vi "Test_Sumadores_Javi.vi"(8 "error in (no error)":errorcluster, 9 "QR":string, 10 "Path":path, 11 "NUMERO DE PASADA DE TEST":i32) -> (0 "Boolean":bool)   [LabVIEW 2019]
uses:
  Estados.ctl
  Global_STOP.vi
  Library VI/Global cuenta erroes.vi
  Viejos/Alfredo LABVIEW/Set-up verificador ASICs/Lib Agilent 81160A/Agilent 81150/Agilent 81150.lvlib
panel:
  out "Errores Asic":i32
  out "CIERRE SESION HANDLE TARJETA":u32(ring) items=["FT_OK", "FT_INVALID_HANDLE", "FT_DEVICE_NOT_FOUND", "FT_DEVICE_NOT_OPENED", "FT_IO_ERROR", "FT_INSUFFICIENT_RESOURCES", "FT_INVALID_PARAMETER", "FT_INVALID_BAUD_RATE", "FT_DEVICE_NOT_OPENED_FOR_ERASE", "FT_DEVICE_NOT_OPENED_FOR_WRITE", "FT_FAILED_TO_WRITE_DEVICE", "FT_EEPROM_READ_FAILED", "FT_EEPROM_WRITE_FAILED", "FT_EEPROM_ERASE_FAILED", "FT_EEPROM_NOT_PRESENT", "FT_EEPROM_NOT_PROGRAMMED", "FT_INVALID_ARGS", "FT_NOT_SUPPORTED", "FT_OTHER_ERROR"]
  out "HANDLE":u32
  out "Error (\"1\" Error)":bool
  out "Todos":T1(array[cluster])=[{"Device Index"=0, "FT_FLAGS_OPENED"=TRUE, "FT_FLAGS_HISPEED"=TRUE, "Type"=6, "VID"=1027, "PID"=24592, "LocID"=1131585, "Serial Number"="CTAV2022A", "Description"="MI CTA TEST A", "FT_Handle"=433820616}, {"Device Index"=1, "FT_FLAGS_OPENED"=TRUE, "FT_FLAGS_HISPEED"=TRUE, "Type"=6, "VID"=1027, "PID"=24592, "LocID"=1131586, "Serial Number"="CTAV2022B", "Description"="MI CTA TEST B", "FT_Handle"=433822896}]
  out "Array CTA":T1(array[cluster])=[{"Device Index"=0, "FT_FLAGS_OPENED"=TRUE, "FT_FLAGS_HISPEED"=TRUE, "Type"=6, "VID"=1027, "PID"=24592, "LocID"=1131585, "Serial Number"="CTAV2022A", "Description"="MI CTA TEST A", "FT_Handle"=433820616}]
  out "VISA resource name":refnum<visa-resource-name>
  out "error out":errorcluster
  out "VISA resource name out":refnum<visa-resource-name>
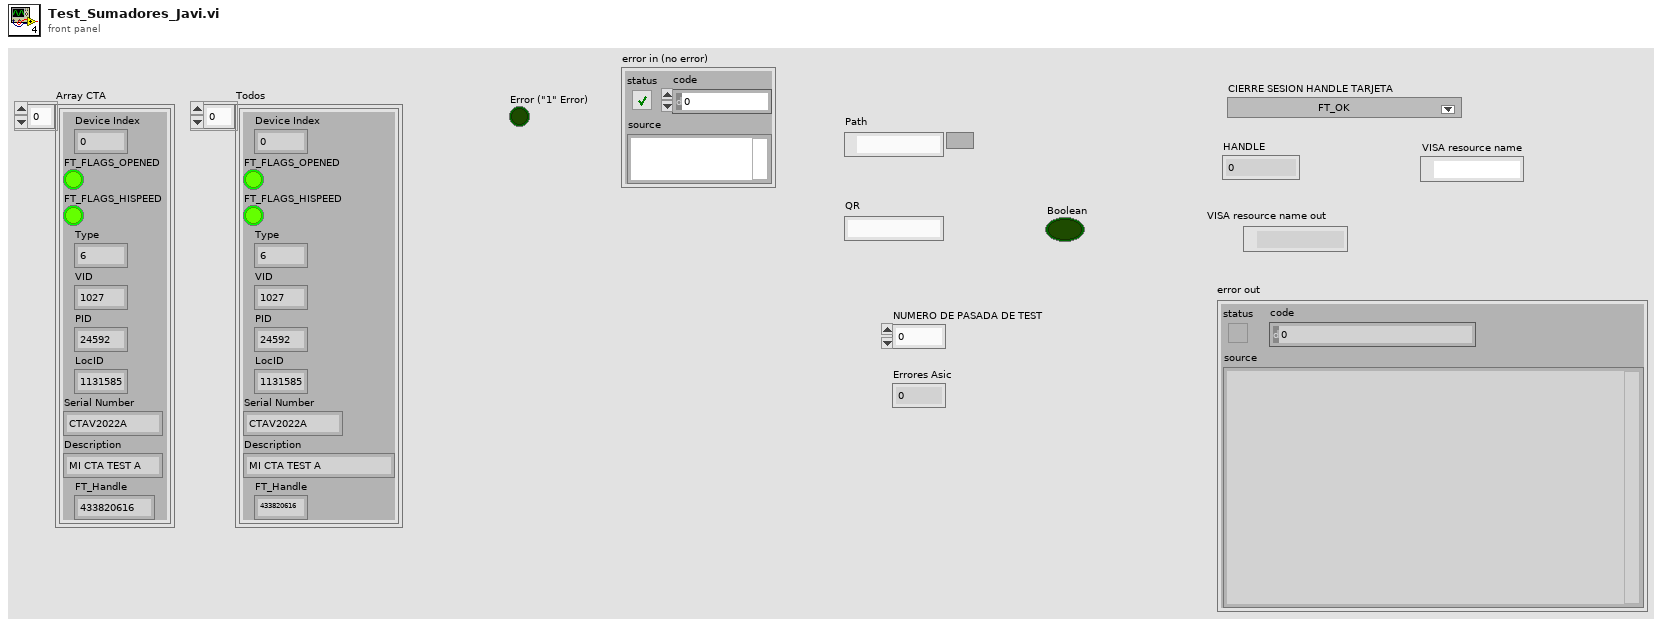
[diagram p1: front panel]
types:
  T1 = cluster{"Device Index":u32, "FT_FLAGS_OPENED":bool, "FT_FLAGS_HISPEED":bool, "Type":u32, "VID":u32, "PID":u32, "LocID":i32, "Serial Number":string, "Description":string, "FT_Handle":u32}[]
  T2 = typedef "Estados.ctl" = enum16{"CrearCabeceraFicheroRegistros", "CreaFicheroRegistros", "Inicio", "FuenteON", "Espera", "FuenteOFF", "ObtenerHandle", "Fin", "RateScan", "CerrarVISA"}
  T3 = typedef "global erroes cluster.ctl" = cluster{"Errores FPGA":i32, "Errores Asic":i32, "Errores ADC adq":i32, "Errores ADC Asic":i32}
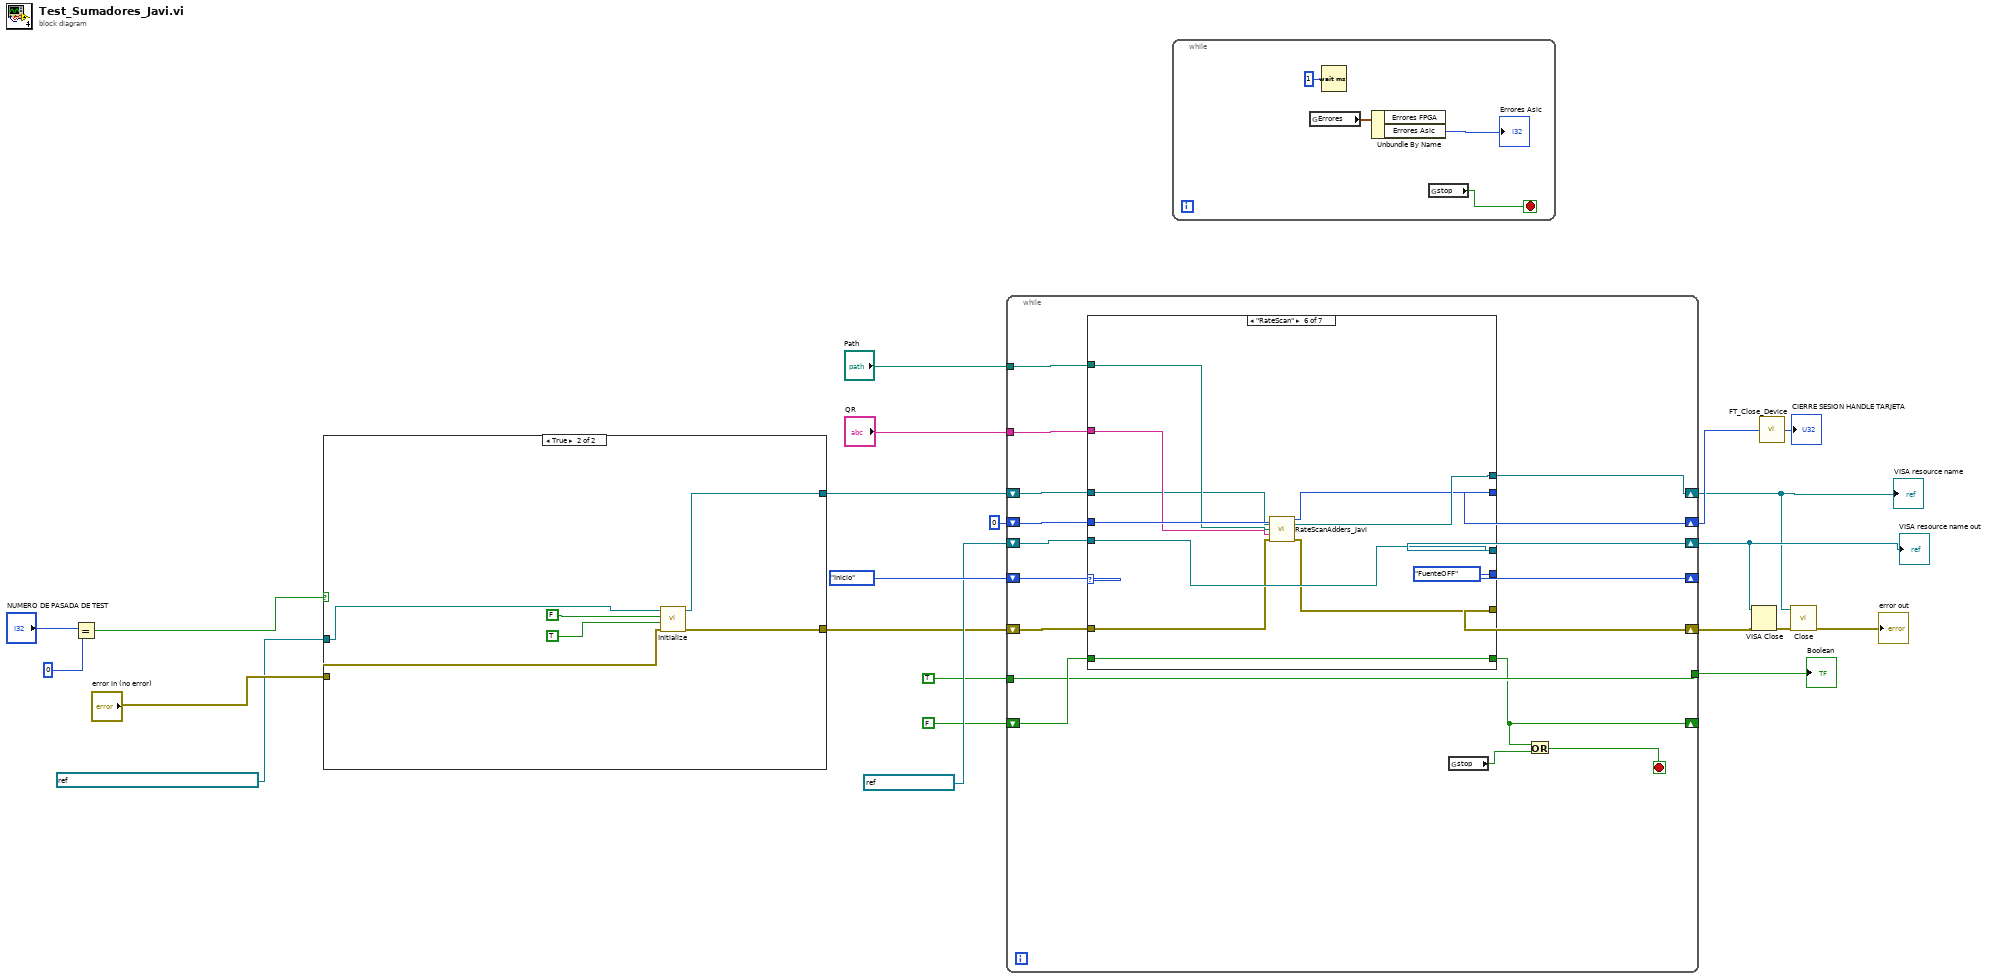
[diagram p0: block diagram]
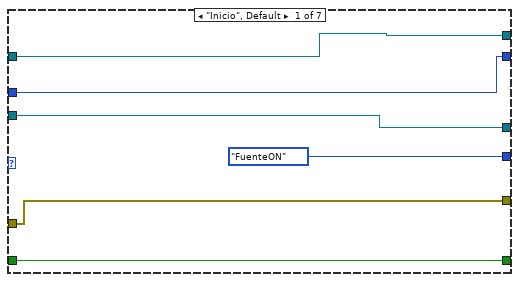
[diagram p3: hidden frame]
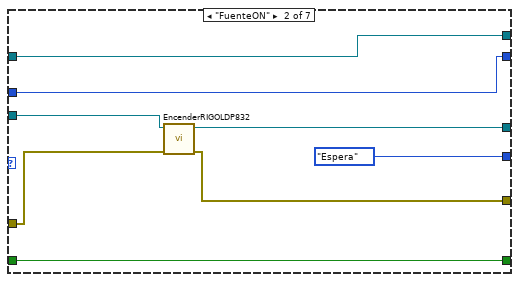
[diagram p4: hidden frame]
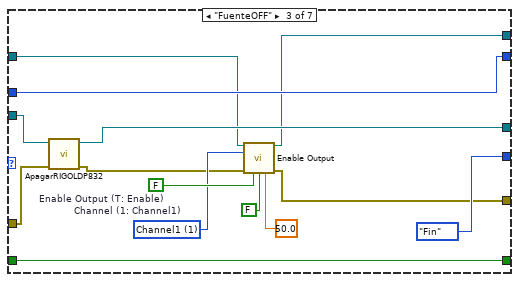
[diagram p5: hidden frame]
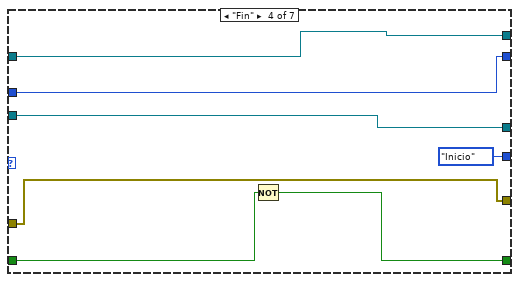
[diagram p6: hidden frame]
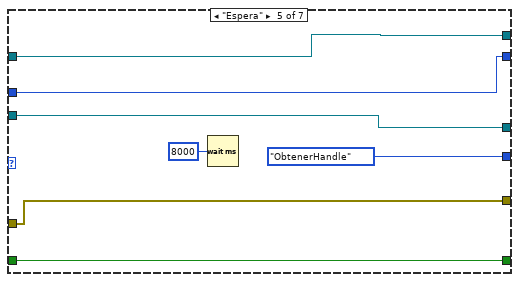
[diagram p7: hidden frame]
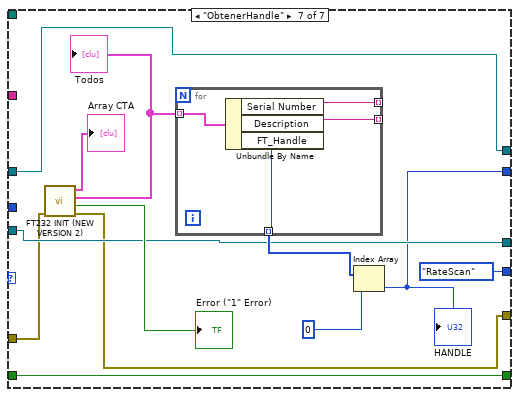
[diagram p8: hidden frame]
diagram:
  n1 = Equal?(x="NUMERO DE PASADA DE TEST", y=0) -> (x = y?=w3:bool)
  n2 = case shown="True" w3 {
    tunnel: [w24 w30] -> w7
    tunnel: [w23 w29] -> w6
    tunnel: "error in (no error)" -> [w24 w28]
    tunnel: refnum<visa-resource-name> "USB0::0x0957::0x4108::MY51400682::INSTR" ("VISA resource name out") -> [w23 w27]
    frame False {
    }
    frame True {
      n3 = call "Initialize.vi"("error in (no error)"=w28, "Reset (True)"=TRUE, "ID Query (True)"=FALSE, "VISA resource name"=w27) -> ("error out"=w30:errorcluster, "VISA resource name out"=w29:refnum<visa-resource-name>)  [unwired: 6 in]
    }
  }
  n4 = while {
    shift-right: [w44] -> _
    shift-left: Estados."Inicio" -> [w47]
    shift-right: [w45] -> w18
    shift-left: refnum<visa-resource-name> "FA_Rigol_DP832" ("VISA IN") -> [w46]
    shift-right: [w37] -> w19
    shift-left: w7 -> [w38]
    shift-right: [w33] -> _
    shift-left: FALSE -> [w43]
    shift-right: [w41] -> w10
    shift-left: w6 -> [w42]
    shift-right: [w40] -> w16
    shift-left: u32 0 ("FT_Handle") -> [w39]
    tunnel: "QR" -> [w36]
    tunnel: "Path" -> [w35]
    tunnel: [w34] -> w11
    tunnel: TRUE -> [w34]
    stop <- w31 stop-if-true
    n5 = case shown="\"RateScan\"" w47 {
      tunnel: [Estados."FuenteON" Estados."Espera" Estados."Fin" Estados."Inicio" Estados."ObtenerHandle" Estados."FuenteOFF" Estados."RateScan"] -> w44
      tunnel: w46 -> [w52 w60 w71 w82 w88 w98 w104]
      tunnel: [w52 w59 w70 w82 w88 w98 w104] -> w45
      tunnel: w43 -> [w51 w58 w74 w81 w86 w99 w106]
      tunnel: [w51 w58 w74 w80 w86 w99 w106] -> w33
      tunnel: w42 -> [w50 w57 w69 w79 w85 w91 w105]
      tunnel: [w50 w57 w63 w79 w85 w97 w105] -> w41
      tunnel: [w49 w56 w73 w78 w84 w95 w103] -> w40
      tunnel: w39 -> [w49 w56 w73 w78 w84 w96 _]
      tunnel: w38 -> [w48 w55 w72 w76 w83 w90 w102]
      tunnel: [w48 w54 w64 w76 w83 w94 w101] -> w37
      tunnel: w36 -> [_ _ _ _ _ w93 _]
      tunnel: w35 -> [_ _ _ _ _ w92 _]
      frame "Inicio", Default {
      }
      frame "FuenteON" {
        n6 = call "EncenderRIGOLDP832.vi"("error in (no error)"=w55, "VISA IN"=w60) -> ("error out"=w54:errorcluster, "VISA resource name out"=w59:refnum<visa-resource-name>)  [unwired: 8 in]
      }
      frame "FuenteOFF" {
        w67 = u16 1 items=["Channel1"=1, "Channel2"=2]  # Channel (1: Channel1)
        w68 = FALSE  # Enable Output (T: Enable)
        n7 = call "ApagarRIGOLDP832.vi"("error in (no error)"=w72, "VISA resource name"=w71) -> ("error out"=w66:errorcluster, "VISA resource name out"=w70:refnum<visa-resource-name>)  [unwired: 8 in]
        n8 = call "Enable Output.vi"("VISA resource name"=w69, "Channel (1: Channel1)"=w67, "error in (no error)"=w66, "Enable Output (T: Enable)"=w68, "Enable Output Complement (T: Enable)"=FALSE, "Load (50 Ohm)"=50.0) -> ("VISA resource name out"=w63:refnum<visa-resource-name>, "error out"=w64:errorcluster)  [unwired: 8 in]
      }
      frame "Fin" {
        n9 = Not(x=w81) -> (.not. x?=w80:bool)
      }
      frame "Espera" {
        n10 = Wait (ms)(milliseconds to wait=u32 8000) -> ()  [unwired: 1 out]
      }
      frame "RateScan" {
        n11 = call "RateScanAdders_Javi.vi"("ftHandle_in"=w96, "VISA resource name"=w91, "Path"=w92, "String"=w93, "error in (no error)"=w90) -> ("ftHandle_out"=w95:u32, "VISA resource name out"=w97:refnum<visa-resource-name>, "error out"=w94:errorcluster)  [unwired: 8 in]
      }
      frame "ObtenerHandle" {
        n12 = call "FT232 INIT (NEW VERSION 2).vi"("error in (no error)"=w102) -> ("error out"=w101:errorcluster, "Error (\"1\" Error)"=→"Error (\"1\" Error)":bool, "Todos"=w111:T1, "Array CTA"=→"Array CTA":T1)  [unwired: 7 in]
        "Todos" <- w111
        n13 = for {
          tunnel: w111 -> [w116] mode=indexing
          tunnel: [w115] -> _ mode=indexing
          tunnel: [w114] -> _ mode=indexing
          tunnel: [w113] -> w112 mode=indexing
          n14 = Unbundle By Name(w116) -> ("Serial Number"=w115:string, "Description"=w114:string, "FT_Handle"=w113:u32)
        }
        n15 = Index Array(array=w112, index=0) -> (element=w103:u32)
        "HANDLE" <- w103
      }
    }
    n16 = global read "Global_STOP.vi" "stop"() -> (w32:bool)
    n17 = Or(x=w33, y=w32) -> (x .or. y?=w31:bool)
  }
  "VISA resource name out" <- w18
  "VISA resource name" <- w10
  "Boolean" <- w11
  n18 = while {
    stop <- w117 stop-if-true
    n19 = global read "Global cuenta erroes.vi" "Errores"() -> (w120:T3)
    n20 = Wait (ms)(milliseconds to wait=u32 1) -> ()  [unwired: 1 out]
    n21 = Unbundle By Name(w120) -> ("Errores Asic"=→"Errores Asic":i32)  [unwired: 1 out]
    n22 = global read "Global_STOP.vi" "stop"() -> (w117:bool)
  }
  n23 = VISA Close(VISA resource name=w18, error in (no error)=w19) -> (error out=w9:errorcluster)
  n24 = call "FT_Close_Device.vi"("Handle"=w16) -> ("FT_Status"=→"CIERRE SESION HANDLE TARJETA":u32)
  n25 = call "Close.vi"("error in (no error)"=w9, "VISA resource name"=w10) -> ("error out"=→"error out":errorcluster)  [unwired: 9 in]
